vi "Multiplication to null operator selection.vi"(11 "Numeric Control":i32) -> (3 "t":i32)   [LabVIEW 2016]
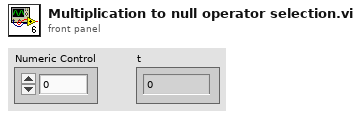
[diagram p1: front panel]
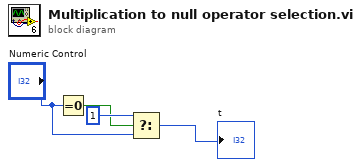
[diagram p0: block diagram]
diagram:
  n1 = Equal To 0?(x="Numeric Control") -> (x = 0?=w1:bool)
  n2 = Select(t=1, s=w1, f="Numeric Control") -> (s? t:f=→"t":i32)
